vi "PD500 - PWM test cleanup.vi"(0 "HMP4040 Channel Settings":T2={"CH1 Voltage"=24.0, "CH1 Current"=1.0, "CH1 Output"=TRUE, "CH2 Voltage"=24.0, "CH2 Current"=1.0, "CH2 Output"=TRUE, "CH3 Voltage"=24.0, "CH3 Current"=1.0, "CH3 Output"=TRUE, "CH4 Voltage"=24.0, "CH4 Current"=1.0, "CH4 Output"=TRUE, "Master Output"=TRUE} {"CH4 Current" format="%.3f"; "CH4 Voltage" format="%.3f"; "CH3 Current" format="%.3f"; "CH3 Voltage" format="%.3f"; "CH2 Current" format="%.3f"; "CH2 Voltage" format="%.3f"; "CH1 Current" format="%.3f"; "CH1 Voltage" format="%.3f"}, 4 "HMP4040_IN":refnum<visa-resource-name>, 6 "Board Selector":T1) -> (12 "T6":dbl[](array[numeric]), 13 "T5":dbl[](array[numeric]), 14 "ControlBoard OUT":refnum<visa-resource-name>, 15 "T4":dbl[](array[numeric]), 16 "T3":dbl[](array[numeric]), 17 "T2":dbl[](array[numeric]), 18 "T1":dbl[](array[numeric]), 19 "error out":errorcluster)   [LabVIEW 2022 SP3]
uses:
  HMP4000 Communication/HMP4040_ChannelControl.ctl
  Serial Board Com/Board Select.ctl
  <vilib>/DAQmx/read.llb/DAQmx Read (Analog 1D Wfm NChan NSamp).vi
  <vilib>/DAQmx/miscellaneous.llb/DAQmx Fill In Error Info.vi
panel:
  out "subarray 12":dbl[](array[numeric])
  out "subarray 11":dbl[](array[numeric])
  out "subarray 10":dbl[](array[numeric])
  out "subarray 9":dbl[](array[numeric])
  out "subarray 8":dbl[](array[numeric])
  out "subarray 7":dbl[](array[numeric])
  out "subarray 6":dbl[](array[numeric])
  out "subarray 5":dbl[](array[numeric])
  out "subarray 4":dbl[](array[numeric])
  out "subarray 3":dbl[](array[numeric])
  out "subarray 2":dbl[](array[numeric])
  out "subarray":dbl[](array[numeric])
  in  "error in (no error) 2":errorcluster
  out "Duty Cycle VISA Write":string[](array[string])
  out "Analysis Leg":i32
  out "Waveforms":T3
  out "Active Leg":i32
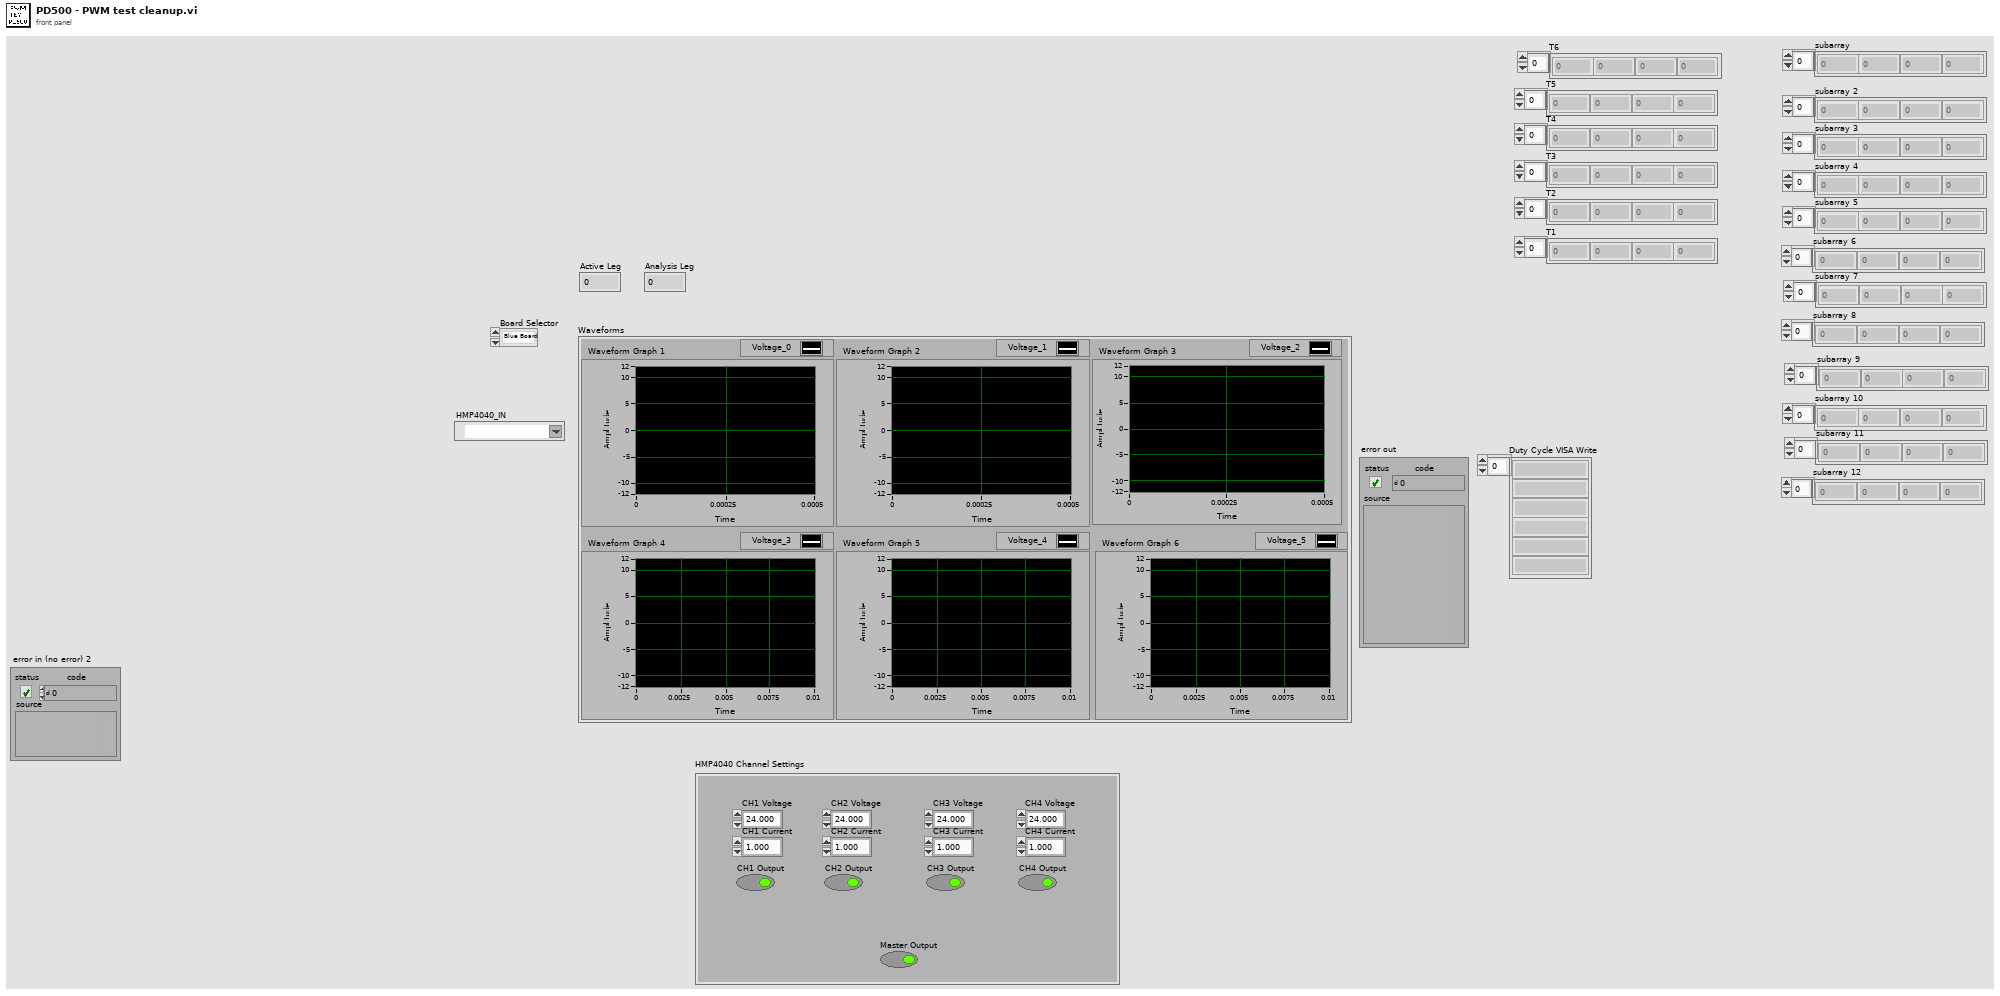
[diagram p1: front panel]
types:
  T1 = typedef "Board Select.ctl" = enum16{"Blue Board", "Green Board"}
  T2 = typedef "HMP4040_ChannelControl.ctl" = cluster{"CH1 Voltage":dbl, "CH1 Current":dbl, "CH1 Output":bool, "CH2 Voltage":dbl, "CH2 Current":dbl, "CH2 Output":bool, "CH3 Voltage":dbl, "CH3 Current":dbl, "CH3 Output":bool, "CH4 Voltage":dbl, "CH4 Current":dbl, "CH4 Output":bool, "Master Output":bool}
  T3 = cluster{"Waveform Graph 1":waveform(dbl), "Waveform Graph 2":waveform(dbl), "Waveform Graph 3":waveform(dbl), "Waveform Graph 4":waveform(dbl), "Waveform Graph 5":waveform(dbl), "Waveform Graph 6":waveform(dbl)}
  T4 = cluster{"data[0]":waveform(dbl), "data[1]":waveform(dbl), "data[2]":waveform(dbl), "data[3]":waveform(dbl), "data[4]":waveform(dbl), "data[5]":waveform(dbl)}
  T5 = typedef "NI_Matrix.lvlib/RealMatrix.ctl" = dbl[][]
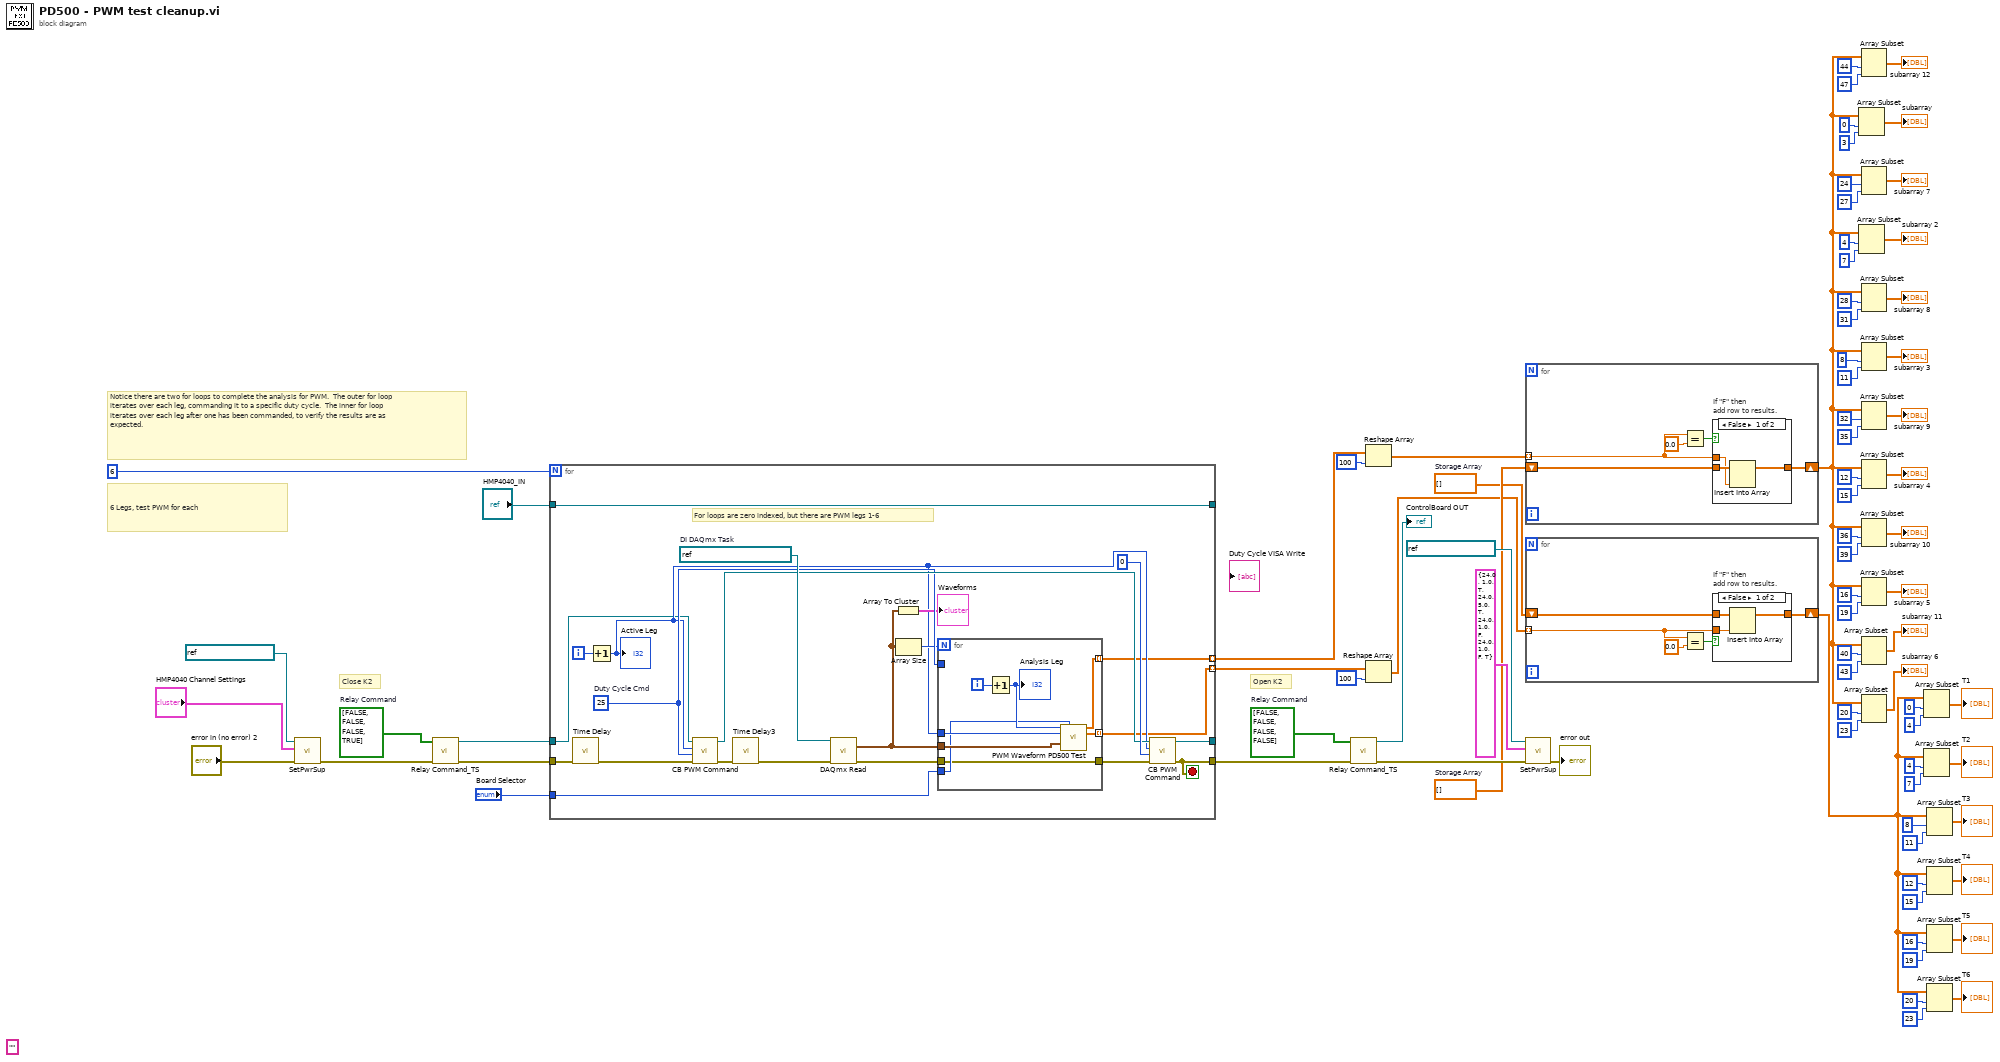
[diagram p0: block diagram]
diagram:
  w58 = dbl[] []  # Storage Array
  w60 = dbl[] []  # Storage Array
  w75 = bool[] [FALSE, FALSE, FALSE, TRUE]  # Relay Command
  w65 = bool[] [FALSE, FALSE, FALSE, FALSE]  # Relay Command
  (unwired) ""
  # "Close K2"
  # "Open K2"
  # "Notice there are two for loops to complete the analysis for PWM.  The outer for loop iterates over each leg, commanding it to a specific duty cycle.  The inner for loop iterates over each leg after one has been commanded, to verify the results are as expected."
  # "6 Legs, test PWM for each"
  n1 = call "SetPwrSup.vi"("error in (no error)"="error in (no error) 2", "HMP4040 Channel Settings"="HMP4040 Channel Settings", "HMP4040 IN"=refnum<visa-resource-name> "HMP4040_FTS2" ("VISA resource name")) -> ("error out"=w71:errorcluster)  [unwired: 7 in, 1 out]
  n2 = call "Relay Command_TS.vi"("error in (no error)"=w71, "Relay Command"=w75) -> ("error out"=w76:errorcluster, "VISA Refnum out"=w78:refnum<visa-resource-name>)  [unwired: 8 in]
  n3 = for {
    N: 6 -> [_]
    tunnel: [w98] -> _
    tunnel: "HMP4040_IN" -> [w98]
    tunnel: [w97] -> w80
    tunnel: [w93] -> _
    tunnel: w76 -> [w87]
    tunnel: w78 -> [w91]
    tunnel: "Board Selector" -> [w88]
    tunnel: [w85] -> w64 mode=indexing
    tunnel: [w84] -> w62 mode=indexing
    i -> [w99]
    stop <- w97 stop-if-true
    w100 = 25  # Duty Cycle Cmd
    w103 = refnum<k21> "FTS2_PWMInput_DG"  # DI DAQmx Task
    # "For loops are zero indexed, but there are PWM legs 1-6"
    n4 = call "Time Delay"("error in (no error)"=w87) -> ("error out"=w86:errorcluster)  [unwired: 10 in]
    n5 = Increment(x=w99) -> (x+1=w92:i32)
    "Active Leg" <- w92
    n6 = call "CB PWM Command.vi"("error in (no error)"=w86, "Duty Cycle"=w100, "Leg"=w92, "VISA Refnum in"=w91) -> ("error out"=w90:errorcluster, "VISA Refnum out"=w101:refnum<visa-resource-name>)  [unwired: 5 in, 1 out]
    n7 = call "Time Delay3"("error in (no error)"=w90) -> ("error out"=w89:errorcluster)  [unwired: 10 in]
    n8 = call-poly <vilib>:"DAQmx Read.vi"("task/channels in"=w103, "error in"=w89) -> ("data"=w94:waveform(dbl)[], "error out"=w82:errorcluster)  [unwired: 11 in, 1 out]
    n9 = Array To Cluster(array=w94) -> (cluster=→"Waveforms":T4)
    n10 = Array Size(array=w94) -> (size(s)=w95:i32)
    n11 = for {
      N: w95 -> [_]
      tunnel: w100 -> [_]
      tunnel: w94 -> [w111]
      tunnel: w92 -> [w110]
      tunnel: w88 -> [w107]
      tunnel: [w106] -> w85 mode=indexing
      tunnel: [w105] -> w84 mode=indexing
      tunnel: [w104] -> w83
      tunnel: w82 -> [w104]
      i -> [w109]
      n12 = Increment(x=w109) -> (x+1=w108:i32)
      "Analysis Leg" <- w108
      n13 = call "PWM Waveform PD500 Test.vi"("Analysis Leg"=w108, "Board Selector"=w107, "Active Leg"=w110, "Waveform"=w111) -> ("Inactive Values"=w106:T5, "Active Values"=w105:T5)  [unwired: 10 in]
    }
    n14 = call "CB PWM Command.vi"("error in (no error)"=w83, "Duty Cycle"=0, "Leg"=w92, "VISA Refnum in"=w101) -> ("error out"=w97:errorcluster, "VISA Refnum out"=w93:refnum<visa-resource-name>)  [unwired: 5 in, 1 out]
  }
  n15 = call "Relay Command_TS.vi"("error in (no error)"=w80, "Relay Command"=w65) -> ("error out"=w68:errorcluster, "VISA Refnum out"=→"ControlBoard OUT":refnum<visa-resource-name>)  [unwired: 8 in]
  n16 = Reshape Array(w64, 100 ("dimension size")) -> (w59:dbl[])
  n17 = Reshape Array(w62, 100 ("dimension size")) -> (w57:dbl[])
  n18 = for {
    tunnel: w59 -> [w114] mode=indexing
    shift-right: [w115] -> w56
    shift-left: w60 -> [w116]
    n19 = Equal?(x=w114, y=0.0) -> (x = y?=w112:bool)
    n20 = case "If \"F\" then \nadd row to results." shown="False" w112 {
      tunnel: w116 -> [w119 w120]
      tunnel: w114 -> [w118 _]
      tunnel: [w117 w120] -> w115
      frame False {
        n21 = Insert Into Array(array=w119, new element=w118) -> (w117:dbl[])  [unwired: 1 in]
      }
      frame True {
      }
    }
  }
  n22 = for {
    tunnel: w57 -> [w123] mode=indexing
    shift-right: [w124] -> w7
    shift-left: w58 -> [w125]
    n23 = Equal?(x=w123, y=0.0) -> (x = y?=w121:bool)
    n24 = case "If \"F\" then \nadd row to results." shown="False" w121 {
      tunnel: w125 -> [w128 w129]
      tunnel: w123 -> [w127 _]
      tunnel: [w126 w129] -> w124
      frame False {
        n25 = Insert Into Array(array=w128, new element=w127) -> (w126:dbl[])  [unwired: 1 in]
      }
      frame True {
      }
    }
  }
  n26 = call "SetPwrSup.vi"("error in (no error)"=w68, "HMP4040 Channel Settings"=T2 {"CH1 Voltage"=24.0, "CH1 Current"=1.0, "CH1 Output"=TRUE, "CH2 Voltage"=24.0, "CH2 Current"=5.0, "CH2 Output"=TRUE, "CH3 Voltage"=24.0, "CH3 Current"=1.0, "CH3 Output"=FALSE, "CH4 Voltage"=24.0, "CH4 Current"=1.0, "CH4 Output"=FALSE, "Master Output"=TRUE}, "HMP4040 IN"=refnum<visa-resource-name> "HMP4040_FTS2" ("VISA resource name")) -> ("error out"=→"error out":errorcluster)  [unwired: 7 in, 1 out]
  n27 = Array Subset(array=w56, index=0, length=3) -> (→"subarray":dbl[])
  n28 = Array Subset(array=w56, index=4, length=7) -> (→"subarray 2":dbl[])
  n29 = Array Subset(array=w56, index=44, length=47) -> (→"subarray 12":dbl[])
  n30 = Array Subset(array=w56, index=24, length=27) -> (→"subarray 7":dbl[])
  n31 = Array Subset(array=w56, index=28, length=31) -> (→"subarray 8":dbl[])
  n32 = Array Subset(array=w56, index=8, length=11) -> (→"subarray 3":dbl[])
  n33 = Array Subset(array=w56, index=32, length=35) -> (→"subarray 9":dbl[])
  n34 = Array Subset(array=w56, index=12, length=15) -> (→"subarray 4":dbl[])
  n35 = Array Subset(array=w56, index=36, length=39) -> (→"subarray 10":dbl[])
  n36 = Array Subset(array=w56, index=16, length=19) -> (→"subarray 5":dbl[])
  n37 = Array Subset(array=w56, index=40, length=43) -> (→"subarray 11":dbl[])
  n38 = Array Subset(array=w56, index=20, length=23) -> (→"subarray 6":dbl[])
  n39 = Array Subset(array=w7, index=0, length=4) -> (→"T1":dbl[])
  n40 = Array Subset(array=w7, index=4, length=7) -> (→"T2":dbl[])
  n41 = Array Subset(array=w7, index=8, length=11) -> (→"T3":dbl[])
  n42 = Array Subset(array=w7, index=12, length=15) -> (→"T4":dbl[])
  n43 = Array Subset(array=w7, index=16, length=19) -> (→"T5":dbl[])
  n44 = Array Subset(array=w7, index=20, length=23) -> (→"T6":dbl[])
